vi "Write Name.vi"(8 "error in (no error)":errorcluster, 10 "Name":string, 11 "Metric in":refnum<class "Metric.lvclass">) -> (0 "error out":errorcluster, 3 "Metric out":refnum<class "Metric.lvclass">)   [LabVIEW 2020, in "Metrics.lvlib" / "Metric.lvclass"]
uses:
  Metric.lvclass
  Metric.lvclass/Metric.ctl
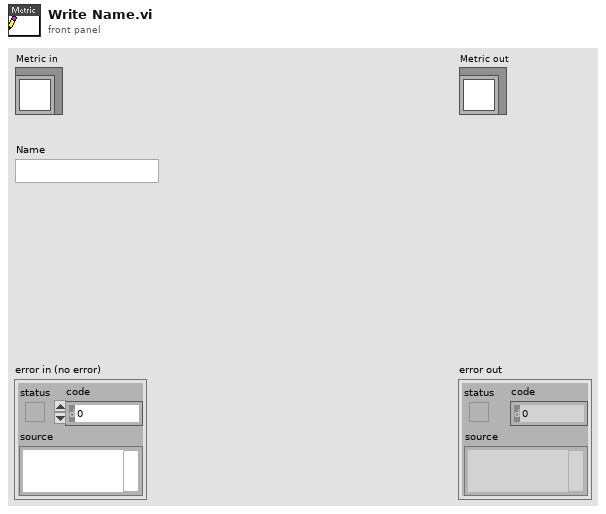
[diagram p1: front panel]
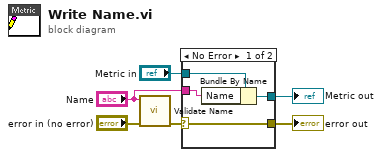
[diagram p0: block diagram]
diagram:
  n1 = call "Validate Name.vi"("error in (no error)"="error in (no error)", "Name"="Name") -> ("error out"=w2:errorcluster)  [unwired: 8 in, 1 out]
  n2 = case shown="No Error" w2 {
    selector: w2 -> [w7 w12]
    tunnel: "Metric in" -> [w10 w11]
    tunnel: [w9 w11] -> w5
    tunnel: "Name" -> [w8 _]
    tunnel: [w7 w12] -> w1
    frame No Error {
      n3 = Bundle By Name(cluster=w10, "Name"=w8) -> (w9:refnum<class "Metric.lvclass">)
    }
    frame Error {
    }
  }
  "error out" <- w1
  "Metric out" <- w5
